vi "ADC_Sweep_Voltage_Gen.vi"(6 "Shuffle":bool, 9 "Count":i32=11, 10 "Vn":dbl=-2.45 format="%#_13g", 11 "Vp":dbl=2.45 format="%#_13g") -> (3 "Vin_Array_Set":dbl[](array[numeric])=[0.05, 0.26818181818181824, 0.48636363636363644, 0.7045454545454547, 0.922727272727273, 1.140909090909091, 1.3590909090909093, 1.5772727272727276, 1.7954545454545459, 2.013636363636364, 2.231818181818182, 2.45])   [LabVIEW 2019]
uses:
  3898d246-1a1b-4163-ae34-6d319fd95c0d.vi
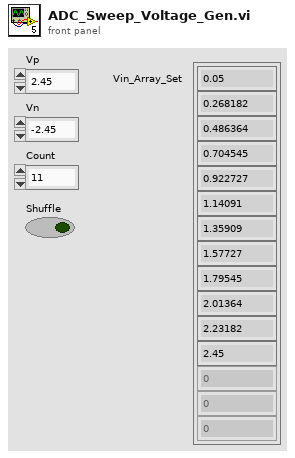
[diagram p1: front panel]
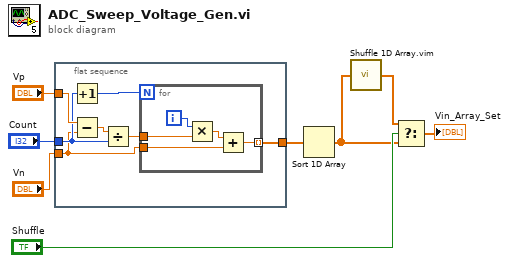
[diagram p0: block diagram]
diagram:
  n1 = flat-sequence {
    tunnel: "Vp" -> [w12]
    tunnel: "Vn" -> [w9]
    tunnel: "Count" -> [w11]
    tunnel: [w10] -> w5
    frame #0 {
      n2 = Increment(x=w11) -> (x+1=w15:i32)
      n3 = Subtract(x=w12, y=w9) -> (x-y=w13:dbl)
      n4 = Divide(x=w13, y=w11) -> (x/y=w14:dbl)
      n5 = for {
        N: w15 -> [_]
        tunnel: w14 -> [w20]
        tunnel: w9 -> [w18]
        tunnel: [w16] -> w10 mode=indexing
        i -> [w19]
        n6 = Multiply(x=w19, y=w20) -> (x*y=w17:dbl)
        n7 = Add(x=w17, y=w18) -> (x+y=w16:dbl)
      }
    }
  }
  n8 = Sort 1D Array(array=w5) -> (sorted array=w2:dbl[])
  n9 = call "Shuffle 1D Array.vim"("array"=w2) -> ("shuffled array"=w1:dbl[])  [unwired: 4 in]
  n10 = Select(t=w1, s="Shuffle", f=w2) -> (s? t:f=→"Vin_Array_Set":dbl[])
